vi "Reset-characteristics-file.vi"(8 "error in (no error)":errorcluster, 11 "Storage params. ref. in":refnum<data-value>) -> (0 "error out":errorcluster, 3 "Storage params. ref.":refnum<data-value>)   [LabVIEW 2013, in "CameraVision.lvlib" / "CV-Storage.lvclass"]
doc: "Check if the characteristics file should be refreshed and perform the refresh if necessary (close the old file reference and open a new file reference using the new file name parameters).\n\nThe file is refreshed if the characteristics have to be saved AND ¦ it is either the first iteration/layer of a new acquisition OR a new file is needed for every iteration/layer within the same acquisition."
uses:
  CV-Storage.lvclass
  CV-Storage.lvclass/CV-Storage.ctl
  UI/Module-states.ctl
  Write Characteristics storage status.vi
  Read Layer index.vi
  Read Storage mode.vi
  UI/CV-UI.lvclass
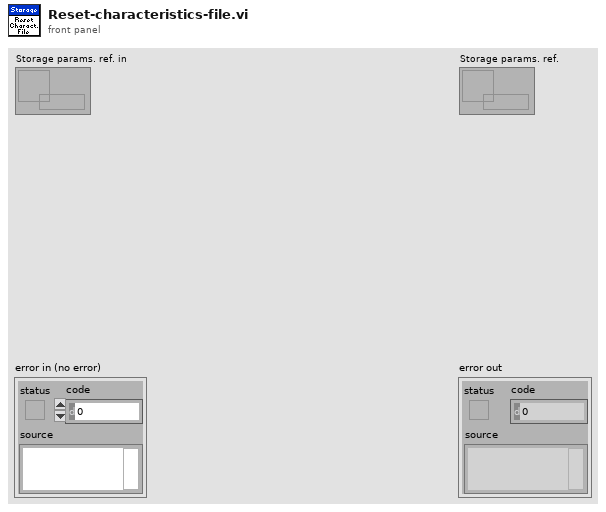
[diagram p1: front panel]
types:
  T1 = enum16{"1 file per layer", "1 file for all layers "}
  T2 = typedef "CameraVision.lvlib/CV-UI.lvclass/Module-states.ctl" = enum16{"Inactive", "Active", "Data-loss", "Error", "Simulation", "Synchronizing", "Initialized", "Released"}
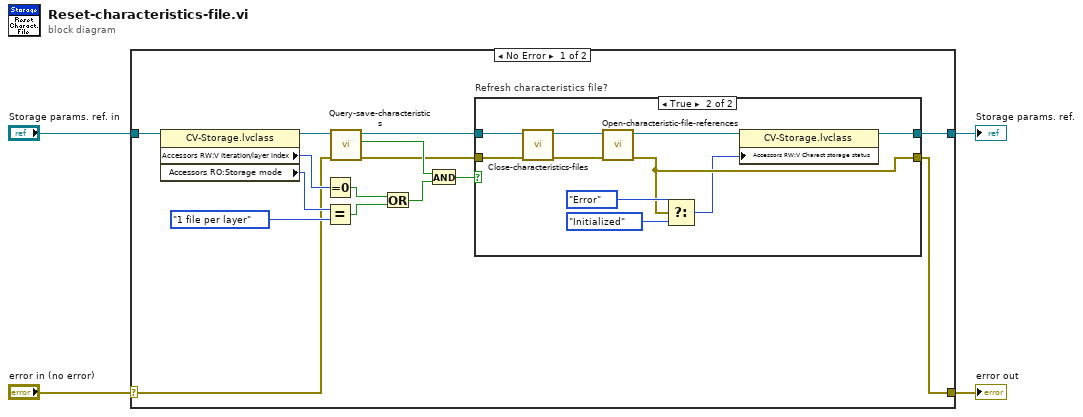
[diagram p0: block diagram]
diagram:
  n1 = case shown="No Error" "error in (no error)" {
    selector: "error in (no error)" -> [w10 w33]
    tunnel: [w6 w33] -> w3
    tunnel: [w5 w32] -> w1
    tunnel: "Storage params. ref. in" -> [w19 w32]
    frame No Error {
      n2 = property class="CV-Storage.lvclass"(reference=w19) -> (reference out=w17:refnum<data-value>, "Accessors RW:V Iteration/layer index"=w18:u16, "Accessors RO:Storage mode"=w14:T1)  [unwired: 1 in, 1 out]
      n3 = Equal To 0?(x=w18) -> (x = 0?=w12:bool)
      n4 = Equal?(x=w14, y=T1."1 file per layer") -> (x = y?=w11:bool)
      n5 = call "Query-save-characteristics.vi"("error in"=w10, "Storage params. ref. in"=w17) -> ("error IO"=w9:errorcluster, "Save characteristics?"=w16:bool, "Storage params. ref."=w8:refnum<data-value>)  [unwired: 7 in]
      n6 = Or(x=w12, y=w11) -> (x .or. y?=w15:bool)
      n7 = And(x=w16, y=w15) -> (x .and. y?=w7:bool)
      n8 = case "Refresh characteristics file?" shown="True" w7 {
        tunnel: w9 -> [w20 w28]
        tunnel: w8 -> [w21 w29]
        tunnel: [w21 w23] -> w5
        tunnel: [w20 w25] -> w6
        frame False {
        }
        frame True {
          n9 = call "Close-characteristics-files.vi"("error in"=w28, "Storage params. ref. in"=w29) -> ("error IO"=w30:errorcluster, "Storage params. ref."=w31:refnum<data-value>)  [unwired: 7 in, 1 out]
          n10 = call "Open-characteristic-file-references.vi"("error in"=w30, "Storage params. ref. in"=w31) -> ("error IO"=w25:errorcluster, "Storage params. ref."=w24:refnum<data-value>)  [unwired: 8 in]
          n11 = Select(t=Module-states."Error" ("Acquisition status"), s=w25, f=Module-states."Initialized" ("Acquisition status")) -> (s? t:f=w22:T2)
          n12 = property class="CV-Storage.lvclass"(reference=w24, "Accessors RW:V Charact storage status"=w22) -> (reference out=w23:refnum<data-value>)  [unwired: 1 in, 1 out]
        }
      }
    }
    frame Error {
    }
  }
  "error out" <- w3
  "Storage params. ref." <- w1
